vi "LVPortGetTempNamepathMap.vi"(9 "Value Type (Or value to update)":variant, 10 "Object ID":i32, 11 "pID":string) -> (3 "Object Map":T1[](array[typedef]))   [LabVIEW 2017]
uses:
  Common/ObjectMap/LVPortObjectMapNamepathData.ctl
  Common/ObjectMap/LVPortObjectMapDataTypeEnum.ctl
  Common/ObjectMap/LVPortObjectMapContainerTypeEnum.ctl
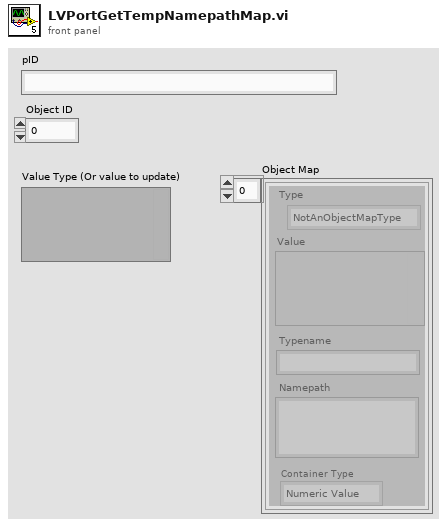
[diagram p1: front panel]
types:
  T1 = typedef "LVPortObjectMapNamepathData.ctl" = cluster{"Type":T2, "Value":variant, "Namepath":string, "Typename":string, "Container Type":T3}
  T2 = typedef "LVPortObjectMapDataTypeEnum.ctl" = enum16{"NotAnObjectMapType", "Real", "Complex", "String", "Boolean"}
  T3 = typedef "LVPortObjectMapContainerTypeEnum.ctl" = enum16{"Numeric Value", "Numeric Array", "Waveform"}
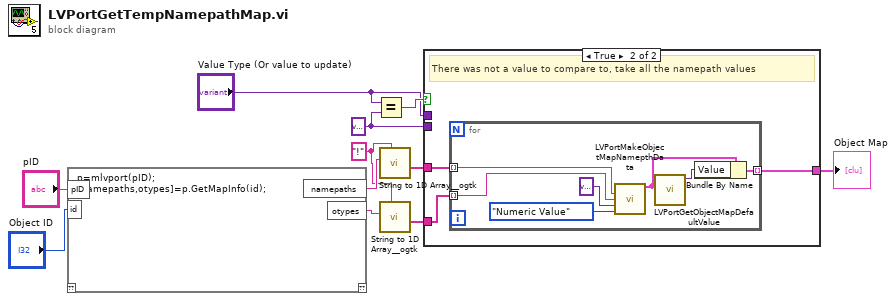
[diagram p0: block diagram]
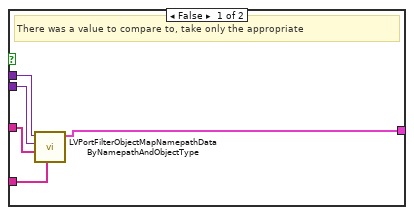
[diagram p2: hidden frame]
diagram:
  w1 = variant
  w7 = "!" ("delimiter (Tab)")
  n1 = script code="p=mlvport(pID);\n[namepaths,otypes]=p.GetMapInfo(id);"("pID"="pID", "id"="Object ID") -> ("namepaths"=w9:string, "otypes"=w8:string)  [unwired: 1 in, 1 out]
  n2 = Equal?(x="Value Type (Or value to update)", y=w1) -> (x = y?=w4:bool)
  n3 = call <userlib>:"String to 1D Array__ogtk.vi"("delimiter (Tab)"=w7, "string"=w9) -> ("Array of Strings"=w6:string[])  [unwired: 9 in]
  n4 = call <userlib>:"String to 1D Array__ogtk.vi"("delimiter (Tab)"=w7, "string"=w8) -> ("Array of Strings"=w5:string[])  [unwired: 9 in]
  n5 = case shown="True" w4 {
    tunnel: w6 -> [w14 w19]
    tunnel: w5 -> [w12 w18]
    tunnel: [w13 w17] -> w3
    tunnel: "Value Type (Or value to update)" -> [w16 _]
    tunnel: w1 -> [w15 _]
    frame False {
      # "There was a value to compare to, take only the appropriate"
      n6 = call "LVPortFilterObjectMapNamepathDataByNamepathAndObjectType.vi"("Object types"=w12, "Namepaths"=w14, "Variant"=w15, "Value Type (Or value to update)"=w16) -> ("ObjectMap"=w13:T1[])  [unwired: 7 in]
    }
    frame True {
      # "There was not a value to compare to, take all the namepath values"
      n7 = for {
        tunnel: w19 -> [w26] mode=indexing
        tunnel: w18 -> [w25] mode=indexing
        tunnel: [w21] -> w17 mode=indexing
        n8 = call "LVPortMakeObjectMapNamepthData.vi"("namepath"=w26, "TypeName"=w25, "value"=variant, "Labview Contriner type"=LVPortObjectMapContainerTypeEnum."Numeric Value") -> ("MatlabDataBundle"=w23:T1)  [unwired: 11 in]
        n9 = call "LVPortGetObjectMapDefaultValue.vi"("Namepath Data in"=w23) -> ("Default Value"=w22:variant)  [unwired: 10 in]
        n10 = Bundle By Name(cluster=w23, "Value"=w22) -> (w21:T1)
      }
    }
  }
  "Object Map" <- w3
